vi "XY Graph Add Single Plot with Name.vi"(0 "XYGraph Ref in":T3, 1 "Scales (Default)":cluster{"X Scale":u32, "Y Scale":u32}, 2 "Plot Interpolation (Previous Plot's Style)":T2=7 items=["Point (.)", "Stepwise Right (--.)", "Line + Point (\\. /)", "Stepwise Left (.--)", "Stepwise Centered (-.-)", "Stepwise Vertical (|.|)", "Line (-)", "Use Previous Plot's Style"], 3 "Keep Existing Plots (T)":bool=TRUE, 5 "Plot":cluster{"X Array":dbl[], "Y Array":dbl[]}, 7 "Plot Metadata":variant, 9 "Plot Name (\"Plot\")":string, 11 "error in (no error)":errorcluster, 13 "Plot Color (Default)":u32(colorbox)=15781887, 14 "Point Style (Dot)":T1=enum."Dot") -> (4 "XY Graph Caption (or Label)":string, 8 "Plot Index":i32, 10 "Plot Name":string, 15 "error out":errorcluster)   [LabVIEW 2019]
uses:
  XY Graph Refnum.ctl
  LabVIEW Plot Interpolation.ctl
  Plot Point Style.ctl
  XY Graph Add-Ons.lvlib
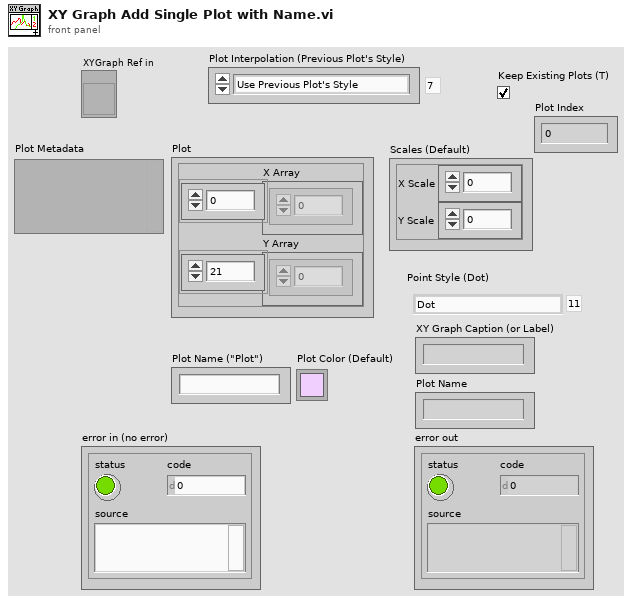
[diagram p1: front panel]
types:
  T1 = typedef "Plot Point Style.ctl" = enum16{"not defined", "None", "Empty Circle", "Filled Circle", "Thick Circle", "Dotted Circle", "Empty Square", "Filled Square", "Thick Square", "Dotted Square", "Small Filled Square", "Dot", "Cross", "Tiny Cross", "Large X", "Small x", "Diamond", "Small Empty Square"}
  T2 = typedef "LabVIEW Plot Interpolation.ctl" = u8
  T3 = typedef "XY Graph Add-Ons.lvlib/XY Graph Refnum.ctl" = refnum<vi>
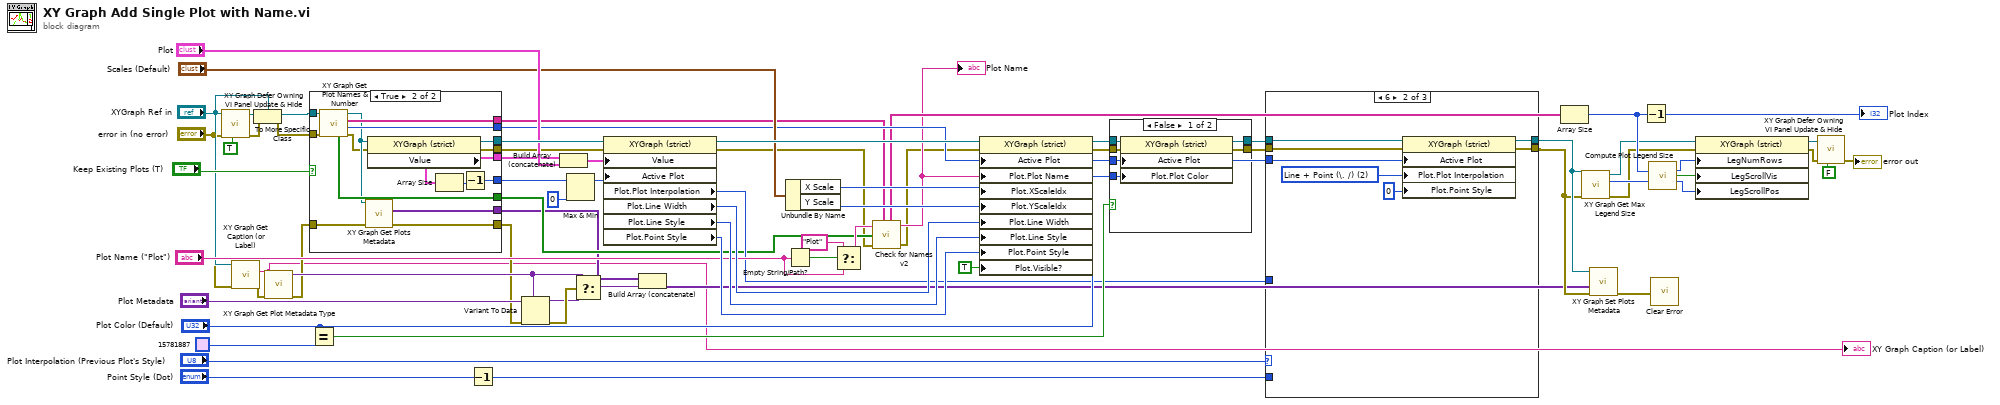
[diagram p0: block diagram]
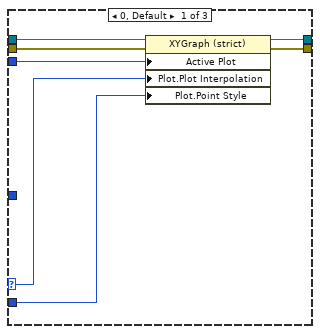
[diagram p3: hidden frame]
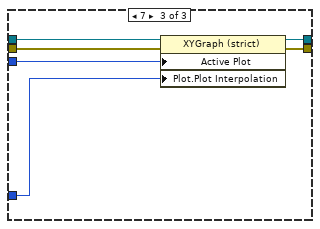
[diagram p4: hidden frame]
diagram:
  n1 = call "XY Graph Defer Owning VI Panel Update & Hide.vi"("Defer Owning Panel Update"=TRUE, "error in (no error)"="error in (no error)", "XY Graph Refnum in"="XYGraph Ref in") -> ("error out"=w28:errorcluster, "XY Graph Refnum out"=w35:refnum<vi>)  [unwired: 7 in]
  n2 = call "XY Graph Get Caption (or Label).vi"("error in (no error)"="error in (no error)", "XYGraph in"="XYGraph Ref in") -> ("error out"=w2:errorcluster, "Caption (or Label) Text"=w1:string)  [unwired: 7 in, 1 out]
  "XY Graph Caption (or Label)" <- w1
  n3 = To More Specific Class(target class="XYGraph Ref in", reference=w35, error in=w28) -> (specific class reference=w29:T3, error out=w27:errorcluster)
  n4 = call "XY Graph Get Plot Metadata Type.vi"("Error In"=w2, "Graph Label"=w1) -> ("Error Out"=w5:errorcluster, "Plot Metadata Type"=w8:variant)  [unwired: 7 in, 1 out]
  n5 = case shown="True" "Keep Existing Plots (T)" {
    tunnel: w29 -> [w75 w90]
    tunnel: [w75 w89] -> w71
    tunnel: w27 -> [w74 w88]
    tunnel: [_ w87] -> w68
    tunnel: [_ w85] -> w67
    tunnel: [_ w84] -> w41
    tunnel: [_ w83] -> w50
    tunnel: [w74 w82] -> w45
    tunnel: [_ w81] -> w32
    tunnel: [_ w78] -> w14
    tunnel: w5 -> [w73 w77]
    tunnel: [w73 w76] -> w4
    frame False {
    }
    frame True {
      n6 = call "XY Graph Get Plot Names & Number.vi"("error in (no error)"=w88, "XYGraph in"=w90) -> ("error out"=w79:errorcluster, "# Plots"=w83:i32, "Plot Names"=w84:string[], "XYGraph out"=w80:T3, "Empty Plots?"=w81:bool[])  [unwired: 5 in]
      n7 = call "XY Graph Get Plots Metadata.vi"("Error In"=w77, "XYGraph Ref"=w80) -> ("Error Out"=w76:errorcluster, "Plots Metadata"=w78:variant[])  [unwired: 6 in, 2 out]
      n8 = property class="XYGraph (strict)"(reference=w80, error in=w79) -> (reference out=w89:T3, error out=w82:errorcluster, "Value"=w87:cluster{"X Array":dbl[], "Y Array":dbl[]}[])
      n9 = Array Size(array=w87) -> (size(s)=w86:i32)
      n10 = Decrement(x=w86) -> (x-1=w85:i32)
    }
  }
  n11 = Equal?(x="Plot Color (Default)", y=u32 15781887 ("Plot Color (Default)")) -> (x = y?=w54:bool)
  n12 = Decrement(x="Point Style (Dot)") -> (x-1=w37:T1)
  n13 = Variant To Data(error in=w4, type=w8, Variant="Plot Metadata") -> (data=w7:variant, error out=w9:errorcluster)
  n14 = Build Array (concatenate)(w68, "Plot") -> (w72:cluster{"X Array":dbl[], "Y Array":dbl[]}[])
  n15 = Max & Min(x=w67, y=0) -> (max(x,y)=w47:i32)  [unwired: 1 out]
  n16 = Select(t=w8, s=w9, f=w7) -> (s? t:f=w6:variant)
  n17 = property class="XYGraph (strict)"(reference=w71, error in=w45, "Value"=w72, "Active Plot"=w47) -> (reference out=w70:T3, error out=w31:errorcluster, "Plot.Plot Interpolation"=w48:u8, "Plot.Line Width"=w66:u8, "Plot.Line Style"=w65:u8, "Plot.Point Style"=w64:u8)
  n18 = Build Array (concatenate)(w14, w6) -> (w13:variant[])
  n19 = Unbundle By Name("Scales (Default)") -> ("X Scale"=w63:u32, "Y Scale"=w62:u32)
  n20 = Empty String/Path?(string/path="Plot Name (\"Plot\")") -> (empty?=w61:bool)
  n21 = Select(t="Plot", s=w61, f="Plot Name (\"Plot\")") -> (s? t:f=w39:string)
  n22 = call "Check for Names v2.vi"("New Name"=w39, "Name List"=w41, "Empty Plots?"=w32, "Error In"=w31) -> ("New Name List"=w40:string[], "New Name"=w38:string, "Error Out"=w30:errorcluster)  [unwired: 2 in, 1 out]
  "Plot Name" <- w38
  n23 = property class="XYGraph (strict)"(reference=w70, error in=w30, "Active Plot"=w50, "Plot.Plot Name"=w38, "Plot.XScaleIdx"=w63, "Plot.YScaleIdx"=w62, "Plot.Line Width"=w66, "Plot.Line Style"=w65, "Plot.Point Style"=w64, "Plot.Visible?"=TRUE ("Plot.Visible")) -> (reference out=w56:T3, error out=w55:errorcluster)
  n24 = case shown="False" w54 {
    tunnel: w56 -> [w96 w98]
    tunnel: [w95 w98] -> w52
    tunnel: w55 -> [w94 w97]
    tunnel: [w93 w97] -> w51
    tunnel: w50 -> [w92 _]
    tunnel: "Plot Color (Default)" -> [w91 _]
    frame False {
      n25 = property class="XYGraph (strict)"(reference=w96, error in=w94, "Active Plot"=w92, "Plot.Plot Color"=w91) -> (reference out=w95:T3, error out=w93:errorcluster)
    }
    frame True {
    }
  }
  n26 = case shown="6" "Plot Interpolation (Previous Plot's Style)" {
    selector: "Plot Interpolation (Previous Plot's Style)" -> [w100 _ _]
    tunnel: w52 -> [w105 w112 w118]
    tunnel: [w104 w111 w117] -> w16
    tunnel: w51 -> [w103 w110 w116]
    tunnel: [w102 w109 w115] -> w15
    tunnel: w50 -> [w101 w108 w114]
    tunnel: w48 -> [_ _ w113]
    tunnel: w37 -> [w99 _ _]
    frame 0, Default {
      n27 = property class="XYGraph (strict)"(reference=w105, error in=w103, "Active Plot"=w101, "Plot.Plot Interpolation"=w100, "Plot.Point Style"=w99) -> (reference out=w104:T3, error out=w102:errorcluster)
    }
    frame 6 {
      w107 = T2 2 items=["Point (.)", "Stepwise Right (--.)", "Line + Point (\\. /)", "Stepwise Left (.--)", "Stepwise Centered (-.-)", "Stepwise Vertical (|.|)", "Line (-)", "Use Previous Plot's Style"] ("Plot Interpolation (Previous Plot's Style)")
      n28 = property class="XYGraph (strict)"(reference=w112, error in=w110, "Active Plot"=w108, "Plot.Plot Interpolation"=w107, "Plot.Point Style"=u8 0) -> (reference out=w111:T3, error out=w109:errorcluster)
    }
    frame 7 {
      n29 = property class="XYGraph (strict)"(reference=w118, error in=w116, "Active Plot"=w114, "Plot.Plot Interpolation"=w113) -> (reference out=w117:T3, error out=w115:errorcluster)
    }
  }
  n30 = Array Size(array=w40) -> (size(s)=w25:i32)
  n31 = call "XY Graph Get Max Legend Size.vi"("Error In"=w15, "XYGraph Refnum"=w16) -> ("Error Out"=w19:errorcluster, "Max Legend Size"=w26:i32, "XYGraph Refnum"=w20:T3)  [unwired: 6 in, 1 out]
  n32 = call "XY Graph Set Plots Metadata.vi"("error in (no error)"=w15, "Plots Metadata"=w13, "XY Graph Refnum"=w16) -> ("error out"=w12:errorcluster)  [unwired: 7 in, 1 out]
  n33 = Decrement(x=w25) -> (x-1=→"Plot Index":i32)
  n34 = call "Compute Plot Legend Size.vi"("# Plots"=w25, "Max Legend Size"=w26) -> ("LegNumRows"=w24:u32, "LegScrollVis"=w23:bool, "LegScrollPos"=w22:u32)  [unwired: 11 in]
  n35 = call "Clear Error.vi"("Error In"=w12) -> ()  [unwired: 8 in, 1 out]
  n36 = property class="XYGraph (strict)"(reference=w20, error in=w19, "LegNumRows"=w24, "LegScrollVis"=w23, "LegScrollPos"=w22) -> (reference out=w17:T3, error out=w33:errorcluster)
  n37 = call "XY Graph Defer Owning VI Panel Update & Hide.vi"("Defer Owning Panel Update"=FALSE, "error in (no error)"=w33, "XY Graph Refnum in"=w17) -> ("error out"=→"error out":errorcluster)  [unwired: 7 in, 1 out]
